vi "Controller Test PS-Filters.vi"() -> ()   [LabVIEW 2011]
uses:
  <vilib>/Platform/TimedLoop/XDataNode/timing_clust.ctl
  <vilib>/Platform/TimedLoop/XDataNode/nitl_modes.ctl
  <vilib>/Platform/TimedLoop/XDataNode/wakeup.ctl
  <vilib>/Utility/file.llb/Read From Spreadsheet File (DBL).vi
  <vilib>/Platform/TimedLoop/XDataNode/loadnilvce.vi
  <vilib>/Platform/TimedLoop/XDataNode/XDataNode.xnode
  <vilib>/Platform/TimedLoop/XDataNode/XDNodeRunTimeDep.lvlib
panel:
  in  "Corrector Filter Coefficients File":path=path "c:/fofb/FPGA Filters/02_SISO/PS-Filter Coefficients.txt"
  in  "Value":fxp<+/-,20,5>
  in  "Corrector Name":string="ACH02"
  in  "stop":bool
  out "Waveform Chart":cluster{dbl, dbl}(graph)
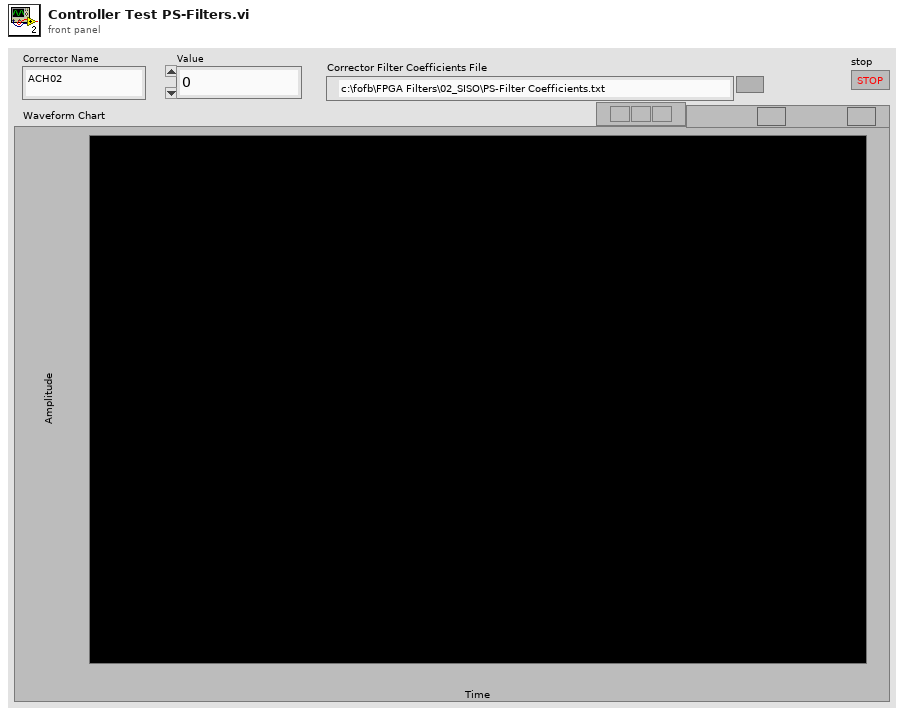
[diagram p1: front panel]
types:
  T1 = typedef "XDNodeRunTimeDep.lvlib/timing_clust.ctl" = cluster{"Expected End [f-1]":u64, "Actual End [f-1]":u64, "Finished Late? [f-1]":bool, "Expected End [i-1]":u64, "Actual End [i-1]":u64, "Finished Late? [i-1]":bool, "Expected Start [i]":u64, "Actual Start [i]":u64, "Expected Start [f]":u64, "Actual Start [f]":u64, "Source Name":string, "Structure Name":string, "Period":i64, "Deadline":i64, "Offset":i64, "Start":i64, "Priority":i32, "Timeout":i32, "Mode":T2, "Wakeup Reason":T3, "Error":errorcluster, "Source Type":string, "Secondary Source Type":string, "Global End Time":u64, "Global Start Time":u64, "Frame Duration":u64, "Iteration Duration":u64, "Assigned CPU":i32, "I/O Scan Engine Mode":u32}
  T2 = typedef "XDNodeRunTimeDep.lvlib/nitl_modes.ctl" = enum32{"No Change", "Process missed periods, maintain original phase", "Discard missed periods, maintain original phase", "Process missed periods, ignore original phase", "Discard missed periods, ignore original phase"}
  T3 = typedef "XDNodeRunTimeDep.lvlib/wakeup.ctl" = enum32{"Normal", "Aborted", "Asynchronous wakeup", "Timing source error", "Timed loop error", "Timeout"}
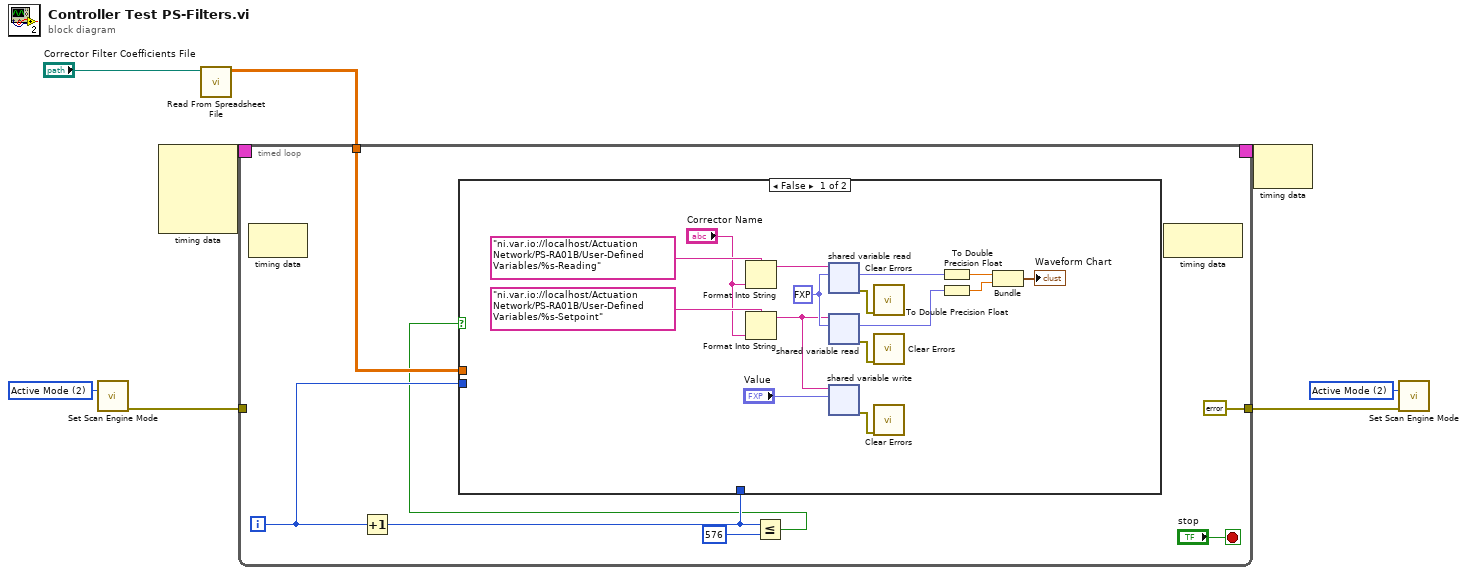
[diagram p0: block diagram]
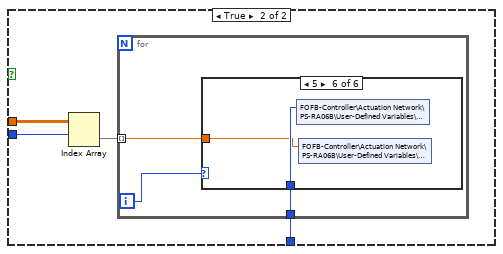
[diagram p2: hidden frame]
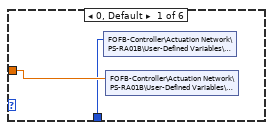
[diagram p3: hidden frame]
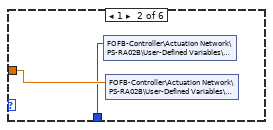
[diagram p4: hidden frame]
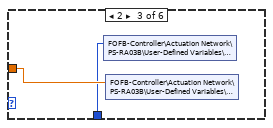
[diagram p5: hidden frame]
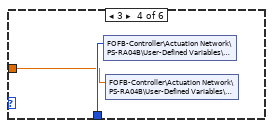
[diagram p6: hidden frame]
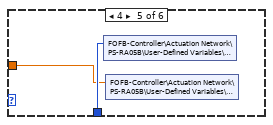
[diagram p7: hidden frame]
diagram:
  w2 = 2 items=["Configuration Mode"=1, "Active Mode"=2] ("mode (Active Mode)")
  w3 = 2 items=["Configuration Mode"=1, "Active Mode"=2] ("mode (Active Mode)")
  n1 = call <vilib>:"Set Scan Engine Mode.vi"("mode (Active Mode)"=w3) -> ("error out"=w4:errorcluster)  [unwired: 14 in]
  n2 = node-c288() -> (w8:T1)  [unwired: 4 in]
  n3 = call-poly <vilib>:"Read From Spreadsheet File.vi"("file path (dialog if empty)"="Corrector Filter Coefficients File") -> ("all rows"=w6:dbl[][])  [unwired: 6 in, 4 out]
  n4 = timed-loop {
    timing: w8 -> [_]
    timing-out: [_] -> w7
    tunnel: w6 -> [w13]
    tunnel: w4 -> [_]
    tunnel: [errorcluster {"status"=FALSE, "code"=0, "source"=""} ("error in (no error)")] -> w1
    i -> [w12]
    stop <- "stop" stop-if-true
    n5 = node-c288() -> ()  [unwired: 1 in, 1 out]
    n6 = Increment(x=w12) -> (x+1=w11:i32)
    n7 = Less Or Equal?(x=w11, y=576) -> (x <= y?=w10:bool)
    n8 = case shown="False" w10 {
      tunnel: w13 -> [_ w34]
      tunnel: w12 -> [_ w33]
      tunnel: w11 -> [_ w31]
      frame False {
        w21 = fxp<+/-,20,5> 0.0 ("data out")
        n9 = Format Into String(format string="ni.var.io://localhost/Actuation Network/PS-RA01B/User-Defined Variables/%s-Reading", "Corrector Name") -> (resulting string=w23:string)  [unwired: 2 in, 1 out]
        n10 = Format Into String(format string="ni.var.io://localhost/Actuation Network/PS-RA01B/User-Defined Variables/%s-Setpoint", "Corrector Name") -> (resulting string=w17:string)  [unwired: 2 in, 1 out]
        n11 = shared-variable-read(w23, w21) -> (w20:errorcluster, w27:fxp<+/-,20,5>)  [unwired: 1 in, 2 out]
        n12 = shared-variable-read(w17, w21) -> (w19:errorcluster, w22:fxp<+/-,20,5>)  [unwired: 1 in, 2 out]
        n13 = shared-variable-write(w17, "Value") -> (w18:errorcluster)  [unwired: 1 in, 1 out]
        n14 = call <vilib>:"Clear Errors.vi"("error in (no error)"=w20) -> ()  [unwired: 6 in, 1 out]
        n15 = call <vilib>:"Clear Errors.vi"("error in (no error)"=w19) -> ()  [unwired: 6 in, 1 out]
        n16 = call <vilib>:"Clear Errors.vi"("error in (no error)"=w18) -> ()  [unwired: 6 in, 1 out]
        n17 = To Double Precision Float(number=w27) -> (double precision float=w28:dbl)
        n18 = To Double Precision Float(number=w22) -> (double precision float=w29:dbl)
        n19 = Bundle(w28, w29) -> (→"Waveform Chart":cluster{dbl, dbl})  [unwired: 1 in]
      }
      frame True {
        n20 = Index Array(array=w34, index (row)=w33) -> (element=w32:dbl[])  [unwired: 1 in]
        n21 = for {
          tunnel: w32 -> [w36] mode=indexing
          tunnel: w31 -> [w35]
          i -> [w37]
          n22 = case shown="5" w37 {
            tunnel: w36 -> [w39 w41 w43 w44 w46 w48]
            tunnel: w35 -> [w38 w40 w42 w45 w47 w49]
            frame 0, Default {
              n23 = shared-variable "FOFB-Controller\\Actuation Network\\PS-RA01B\\User-Defined Variables\\PS-RA01B-ADDR"(w38) -> ()  [unwired: 1 in, 1 out]
              n24 = shared-variable "FOFB-Controller\\Actuation Network\\PS-RA01B\\User-Defined Variables\\PS-RA01B-DATA"(w39) -> ()  [unwired: 1 in, 1 out]
            }
            frame 1 {
              n25 = shared-variable "FOFB-Controller\\Actuation Network\\PS-RA02B\\User-Defined Variables\\PS-RA02B-ADDR"(w40) -> ()  [unwired: 1 in, 1 out]
              n26 = shared-variable "FOFB-Controller\\Actuation Network\\PS-RA02B\\User-Defined Variables\\PS-RA02B-DATA"(w41) -> ()  [unwired: 1 in, 1 out]
            }
            frame 2 {
              n27 = shared-variable "FOFB-Controller\\Actuation Network\\PS-RA03B\\User-Defined Variables\\PS-RA03B-ADDR"(w42) -> ()  [unwired: 1 in, 1 out]
              n28 = shared-variable "FOFB-Controller\\Actuation Network\\PS-RA03B\\User-Defined Variables\\PS-RA03B-DATA"(w43) -> ()  [unwired: 1 in, 1 out]
            }
            frame 3 {
              n29 = shared-variable "FOFB-Controller\\Actuation Network\\PS-RA04B\\User-Defined Variables\\PS-RA04B-ADDR"(w45) -> ()  [unwired: 1 in, 1 out]
              n30 = shared-variable "FOFB-Controller\\Actuation Network\\PS-RA04B\\User-Defined Variables\\PS-RA04B-DATA"(w44) -> ()  [unwired: 1 in, 1 out]
            }
            frame 4 {
              n31 = shared-variable "FOFB-Controller\\Actuation Network\\PS-RA05B\\User-Defined Variables\\PS-RA05B-ADDR"(w47) -> ()  [unwired: 1 in, 1 out]
              n32 = shared-variable "FOFB-Controller\\Actuation Network\\PS-RA05B\\User-Defined Variables\\PS-RA05B-DATA"(w46) -> ()  [unwired: 1 in, 1 out]
            }
            frame 5 {
              n33 = shared-variable "FOFB-Controller\\Actuation Network\\PS-RA06B\\User-Defined Variables\\PS-RA06B-ADDR"(w49) -> ()  [unwired: 1 in, 1 out]
              n34 = shared-variable "FOFB-Controller\\Actuation Network\\PS-RA06B\\User-Defined Variables\\PS-RA06B-DATA"(w48) -> ()  [unwired: 1 in, 1 out]
            }
          }
        }
      }
    }
    n35 = node-c288() -> ()  [unwired: 1 in, 1 out]
  }
  n36 = node-c288(w7) -> ()  [unwired: 1 out]
  n37 = call <vilib>:"Set Scan Engine Mode.vi"("mode (Active Mode)"=w2, "error in (no error)"=w1) -> ()  [unwired: 13 in, 1 out]
